vi "subvi_write_to_file.vi"(8 "file (use dialog) in":path, 10 "Analyser2":i32, 11 "Analyser 1":i32) -> ()   [LabVIEW 2014]
uses:
  <vilib>/Utility/file.llb/Write To Spreadsheet File (string).vi
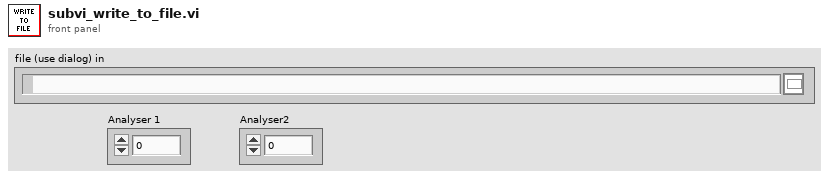
[diagram p1: front panel]
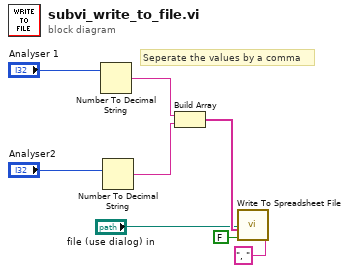
[diagram p0: block diagram]
diagram:
  # "Seperate the values by a comma"
  n1 = Number To Decimal String(number="Analyser 1") -> (decimal integer string=w6:string)  [unwired: 1 in]
  n2 = Number To Decimal String(number="Analyser2") -> (decimal integer string=w7:string)  [unwired: 1 in]
  n3 = Build Array(w6, w7) -> (w8:string[])
  n4 = call-poly <vilib>:"Write To Spreadsheet File.vi"("delimiter (\\t)"=", " ("delimiter (\\t)"), "append to file? (new file:F)"=FALSE, "1D data"=w8, "file path (dialog if empty)"="file (use dialog) in") -> ()  [unwired: 4 in, 1 out]
